vi "Inspect Modules.vi"(7 "Console Log in":refnum<class "Console Log.lvclass">, 8 "error in":errorcluster, 11 "Potting Procedure in":refnum<class "Potting Procedure.lvclass">) -> (0 "error out":errorcluster, 3 "Potting Procedure out":refnum<class "Potting Procedure.lvclass">, 5 "Console Log out":refnum<class "Console Log.lvclass">)   [LabVIEW 2011, in "Potting Procedure.lvclass"]
uses:
  Potting Procedure.lvclass
  UI Classes/Console Log/Console Log.lvclass
  Type Definitions/Inspect Modules.ctl
  Type Definitions/Inspect Modules - Module.ctl
  Shared Components/Utils/Type Definitions/Multi-Fiducial Image.ctl
  Shared Components/Utils/Type Definitions/Physical Image.ctl
  Shared Components/Vec3d Class/Vec3d Class.lvclass
  <vilib>/vision/Image Controls.llb/IMAQ Image.ctl
  Shared Components/Utils/Type Definitions/Fiducial with Source.ctl
  Shared Components/Utils/Type Definitions/Fiducial Image.ctl
  Shared Components/Gantry Class/Gantry Class.lvclass
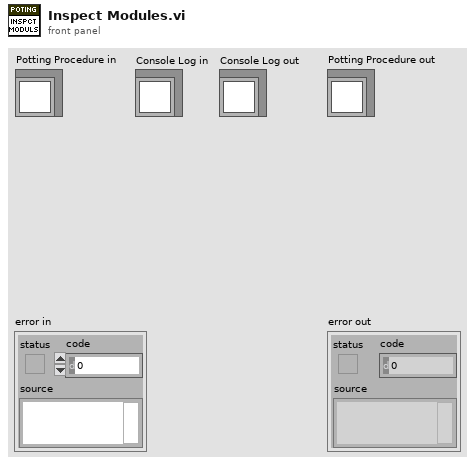
[diagram p1: front panel]
types:
  T1 = typedef "Inspect Modules.ctl" = cluster{"Has Been Run?":bool, "Module Positions":T2[]}
  T2 = typedef "Inspect Modules - Module.ctl" = cluster{"TBM-TBM":T3, "TBM-HDI":T3, "Address Pads":T3, "HDI Bond Pad References":T7[], "BBM Bond Pad References":T7[], "HV-HDI":T7, "HV-BBM":T7, "Chuck":i32, "Slot":i32, "Potting Selection":cluster{"HDI Bond Pads":bool[], "BBM Bond Pads":bool[], "TBM Inner":cluster{"Top":bool, "Left":bool, "Bottom":bool, "Right":bool}, "TBM Outer":cluster{"Top":bool, "Left":bool, "Bottom":bool, "Right":bool}, "Address Pads":cluster{"Top":bool, "Bottom":bool}, "High Voltage":cluster{"HDI":bool, "Sensor":bool}}}
  T3 = typedef "Multi-Fiducial Image.ctl" = cluster{"Fiducial Image":T4, "Fiducials":cluster{"Selected Fiducial":T6, "fiducial name":string}[]}
  T4 = typedef "Physical Image.ctl" = cluster{"Image Position":refnum<class "Vec3d Class.lvclass">, "Image Reference":T5, "Field of View":cluster{"x(mm)":dbl, "y(mm)":dbl}}
  T5 = typedef "IMAQ Image.ctl" = refnum<image>
  T6 = typedef "Fiducial with Source.ctl" = cluster{"Fiducial Image Coordinate":refnum<class "Vec3d Class.lvclass">, "Fiducial Source":enum16{"Pattern Recognition", "User", "Error", "Default"}}
  T7 = typedef "Fiducial Image.ctl" = cluster{"Fiducial Image":T4, "Selected Fiducial":T6, "fiducial name":string}
  T8 = typedef "Inspect Fiducials.ctl" = cluster{"Has Been Run?":bool, "Module-Chuck Fiducials":cluster{"Fiducials-HDI":T7[], "Fiducials-BBM":T7[], "Chuck":i32, "Slot":i32}[]}
  T9 = cluster{"Fiducials-HDI":T7[], "Fiducials-BBM":T7[], "Chuck":i32, "Slot":i32}[]
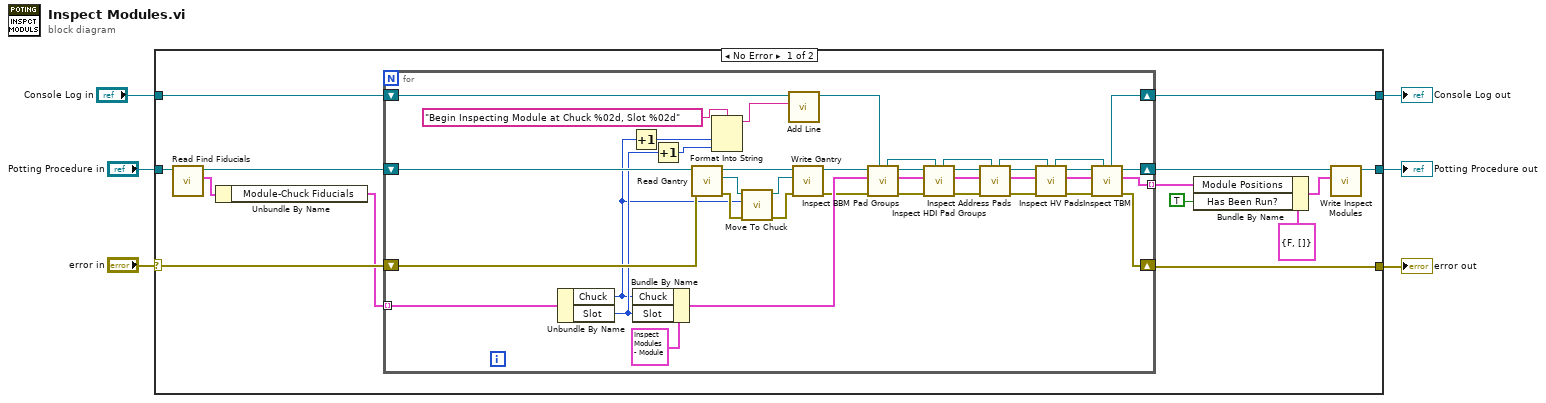
[diagram p0: block diagram]
diagram:
  n1 = case shown="No Error" "error in" {
    selector: "error in" -> [w20 w63]
    tunnel: [w19 w63] -> w5
    tunnel: [w13 w62] -> w3
    tunnel: "Potting Procedure in" -> [w18 w62]
    tunnel: "Console Log in" -> [w8 w61]
    tunnel: [w7 w61] -> w1
    frame No Error {
      n2 = call-dynamic "Read Find Fiducials.vi"("Potting Procedure in"=w18) -> ("Find Fiducials"=w16:T8, "Potting Procedure out"=w17:refnum<class "Potting Procedure.lvclass">)  [unwired: 8 in, 1 out]
      n3 = Unbundle By Name(w16) -> ("Module-Chuck Fiducials"=w15:T9)
      n4 = for {
        shift-right: [w60] -> w14
        shift-left: w17 -> [w41]
        shift-right: [w59] -> w19
        shift-left: w20 -> [w40]
        tunnel: w15 -> [w58] mode=indexing
        tunnel: [w45] -> w9 mode=indexing
        shift-right: [w30] -> w7
        shift-left: w8 -> [w29]
        n5 = Unbundle By Name(w58) -> ("Chuck"=w21:i32, "Slot"=w25:i32)
        n6 = Increment(x=w21) -> (x+1=w23:i32)
        n7 = Bundle By Name(cluster=T2 {"TBM-TBM"={"Fiducial Image"={"Image Position"=refnum, "Image Reference"=refnum, "Field of View"={"x(mm)"=0.0, "y(mm)"=0.0}}, "Fiducials"=[]}, "TBM-HDI"={"Fiducial Image"={"Image Position"=refnum, "Image Reference"=refnum, "Field of View"={"x(mm)"=0.0, "y(mm)"=0.0}}, "Fiducials"=[]}, "Address Pads"={"Fiducial Image"={"Image Position"=refnum, "Image Reference"=refnum, "Field of View"={"x(mm)"=0.0, "y(mm)"=0.0}}, "Fiducials"=[]}, "HDI Bond Pad References"=[], "BBM Bond Pad References"=[], "HV-HDI"={"Fiducial Image"={"Image Position"=refnum, "Image Reference"=refnum, "Field of View"={"x(mm)"=0.0, "y(mm)"=0.0}}, "Selected Fiducial"={"Fiducial Image Coordinate"=refnum, "Fiducial Source"=enum."Pattern Recognition"}, "fiducial name"=""}, "HV-BBM"={"Fiducial Image"={"Image Position"=refnum, "Image Reference"=refnum, "Field of View"={"x(mm)"=0.0, "y(mm)"=0.0}}, "Selected Fiducial"={"Fiducial Image Coordinate"=refnum, "Fiducial Source"=enum."Pattern Recognition"}, "fiducial name"=""}, "Chuck"=0, "Slot"=0, "Potting Selection"={"HDI Bond Pads"=[TRUE, TRUE, TRUE, TRUE, TRUE, TRUE, TRUE, TRUE, TRUE, TRUE, TRUE, TRUE, TRUE, TRUE, TRUE, TRUE], "BBM Bond Pads"=[TRUE, TRUE, TRUE, TRUE, TRUE, TRUE, TRUE, TRUE, TRUE, TRUE, TRUE, TRUE, TRUE, TRUE, TRUE, TRUE], "TBM Inner"={"Top"=TRUE, "Left"=TRUE, "Bottom"=TRUE, "Right"=TRUE}, "TBM Outer"={"Top"=TRUE, "Left"=TRUE, "Bottom"=TRUE, "Right"=TRUE}, "Address Pads"={"Top"=TRUE, "Bottom"=TRUE}, "High Voltage"={"HDI"=TRUE, "Sensor"=TRUE}}} ("Module"), "Chuck"=w21, "Slot"=w25) -> (w44:T2)
        n8 = Increment(x=w25) -> (x+1=w24:i32)
        n9 = call-dynamic "Read Gantry.vi"("error in (no error)"=w40, "Potting Procedure in"=w41) -> ("error out"=w43:errorcluster, "Gantry"=w42:refnum<class "Gantry Class.lvclass">, "Potting Procedure out"=w37:refnum<class "Potting Procedure.lvclass">)  [unwired: 7 in]
        n10 = Format Into String(format string="Begin Inspecting Module at Chuck %02d, Slot %02d" ("initial string"), w23, w24) -> (resulting string=w27:string)  [unwired: 2 in, 1 out]
        n11 = call-dynamic "Move To Chuck.vi"("error in"=w43, "Chuck"=w21, "Gantry in"=w42) -> ("error out"=w39:errorcluster, "Gantry out"=w38:refnum<class "Gantry Class.lvclass">)  [unwired: 7 in]
        n12 = call "Add Line.vi"("String"=w27, "Console Log in"=w29) -> ("Console Log out"=w28:refnum<class "Console Log.lvclass">)  [unwired: 8 in, 1 out]
        n13 = call-dynamic "Write Gantry.vi"("error in (no error)"=w39, "Gantry"=w38, "Potting Procedure in"=w37) -> ("error out"=w35:errorcluster, "Potting Procedure out"=w36:refnum<class "Potting Procedure.lvclass">)  [unwired: 7 in]
        n14 = call-dynamic "Inspect BBM Pad Groups.vi"("Console Log in"=w28, "error in"=w35, "Module Data In"=w44, "Potting Procedure in"=w36) -> ("error out"=w56:errorcluster, "Module Data Out"=w49:T2, "Potting Procedure out"=w57:refnum<class "Potting Procedure.lvclass">, "Console Log out"=w34:refnum<class "Console Log.lvclass">)  [unwired: 4 in]
        n15 = call "Inspect HDI Pad Groups.vi"("Console Log in"=w34, "error in"=w56, "Module Data In"=w49, "Potting Procedure in"=w57) -> ("error out"=w52:errorcluster, "Module Data Out"=w48:T2, "Potting Procedure out"=w55:refnum<class "Potting Procedure.lvclass">, "Console Log out"=w33:refnum<class "Console Log.lvclass">)  [unwired: 4 in]
        n16 = call "Inspect Address Pads.vi"("Console Log in"=w33, "error in"=w52, "Module Data In"=w48, "Potting Procedure in"=w55) -> ("error out"=w51:errorcluster, "Module Data Out"=w47:T2, "Potting Procedure out"=w54:refnum<class "Potting Procedure.lvclass">, "Console Log out"=w32:refnum<class "Console Log.lvclass">)  [unwired: 4 in]
        n17 = call "Inspect HV Pads.vi"("Console Log in"=w32, "error in"=w51, "Module Data In"=w47, "Potting Procedure in"=w54) -> ("error out"=w50:errorcluster, "Module Data Out"=w46:T2, "Potting Procedure out"=w53:refnum<class "Potting Procedure.lvclass">, "Console Log out"=w31:refnum<class "Console Log.lvclass">)  [unwired: 4 in]
        n18 = call "Inspect TBM.vi"("Console Log in"=w31, "error in"=w50, "Module Data In"=w46, "Potting Procedure in"=w53) -> ("error out"=w59:errorcluster, "Module Data Out"=w45:T2, "Potting Procedure out"=w60:refnum<class "Potting Procedure.lvclass">, "Console Log out"=w30:refnum<class "Console Log.lvclass">)  [unwired: 4 in]
      }
      n19 = Bundle By Name(cluster=T1 {"Has Been Run?"=FALSE, "Module Positions"=[]} ("Inspect Modules"), "Module Positions"=w9, "Has Been Run?"=TRUE) -> (w11:T1)
      n20 = call-dynamic "Write Inspect Modules.vi"("Inspect Modules"=w11, "Potting Procedure in"=w14) -> ("Potting Procedure out"=w13:refnum<class "Potting Procedure.lvclass">)  [unwired: 8 in, 1 out]
    }
    frame Error {
    }
  }
  "error out" <- w5
  "Potting Procedure out" <- w3
  "Console Log out" <- w1
